vi "Collect SM Refs.vi"(8 "error in (no error)":errorcluster, 11 "Refs In":T1) -> (0 "error out":errorcluster, 3 "Refs":T1)   [LabVIEW 2022 SP3, in "FlexBlocks Support.lvlib"]
uses:
  FlexBlocks Support.lvlib
  SM Refs.ctl
  <vilib>/Utility/traverseref.llb/TRef TravTarget.ctl
  9901a224-97aa-422c-b79c-d7e7d68877ba.vi
  SM Ref Taversal Callback.vi
  <vilib>/Utility/traverseref.llb/Traverse for GObjects.vi
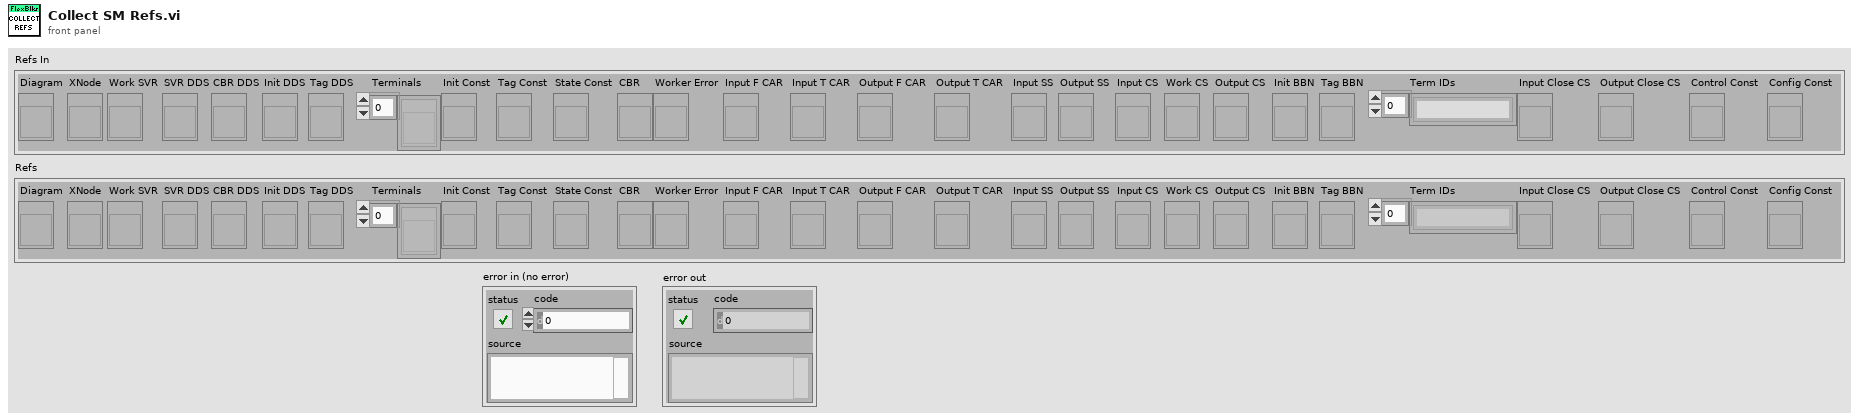
[diagram p1: front panel]
types:
  T1 = typedef "FlexBlocks Support.lvlib/SM Refs.ctl" = cluster{"Diagram":refnum<vi>, "XNode":refnum<vi>, "Work SVR":refnum<vi>, "SVR DDS":refnum<vi>, "CBR DDS":refnum<vi>, "Init DDS":refnum<vi>, "Tag DDS":refnum<vi>, "Terminals":refnum<vi>[], "Init Const":refnum<vi>, "Tag Const":refnum<vi>, "State Const":refnum<vi>, "CBR":refnum<vi>, "Worker Error":refnum<vi>, "Input F CAR":refnum<vi>, "Input T CAR":refnum<vi>, "Output F CAR":refnum<vi>, "Output T CAR":refnum<vi>, "Input SS":refnum<vi>, "Output SS":refnum<vi>, "Input CS":refnum<vi>, "Work CS":refnum<vi>, "Output CS":refnum<vi>, "Init BBN":refnum<vi>, "Tag BBN":refnum<vi>, "Term IDs":string[], "Input Close CS":refnum<vi>, "Output Close CS":refnum<vi>, "Control Const":refnum<vi>, "Config Const":refnum<vi>}
  T2 = typedef "TRef TravTarget.ctl" = enum16{"FP", "BD", "Other"}
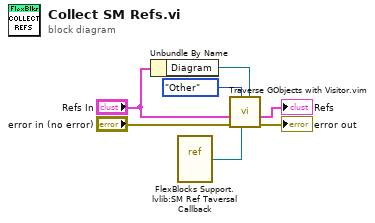
[diagram p0: block diagram]
diagram:
  n1 = Unbundle By Name("Refs In") -> ("Diagram"=w7:refnum<vi>)
  n2 = vi-ref "FlexBlocks Support.lvlib:SM Ref Taversal Callback.vi"() -> (w3:refnum<vi>)
  n3 = call "Traverse GObjects with Visitor.vim"("Other Refnum"=w7, "Visitor VI"=w3, "Traverse Target"=TRef_TravTarget."Other", "error in (no error)"="error in (no error)", "State in"="Refs In") -> ("error out"=→"error out":errorcluster, "State"=→"Refs":T1)  [unwired: 4 in, 1 out]
